vi "SetCurrentLimit.vi"(8 "error in (no error)":errorcluster, 9 "Current":dbl, 10 "Preset":enum16{"0", "1", "2", "3", ""}(ring), 11 "VISA resource name":refnum<visa-resource-name>) -> (0 "error out":errorcluster, 3 "VISA resource name out":refnum<visa-resource-name>)   [LabVIEW 2019, in "9103Series.lvlib"]
doc: "Set the output current limit of the power supply.\n\nPreset: Defines which preset memory to set.\nPreset Values: 3 - Default, 0 - A, 1 - B, 2 - C"
uses:
  <instrlib>/9103Series/9103Series.lvlib
panel:
  out "ok?":string
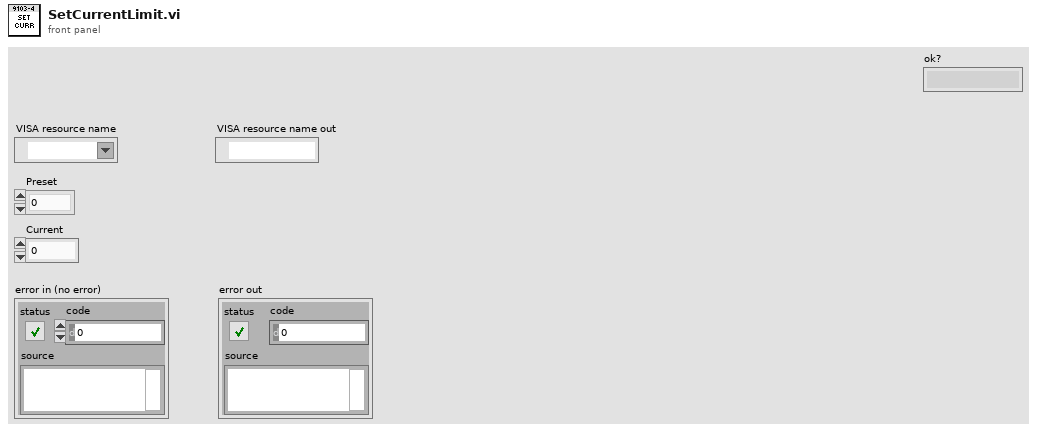
[diagram p1: front panel]
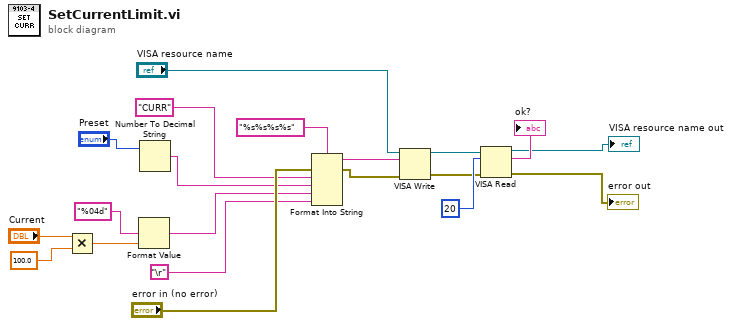
[diagram p0: block diagram]
diagram:
  n1 = Multiply(x="Current", y=100.0) -> (x*y=w17:dbl)
  n2 = Format Value(format string="%04d", value (0)=w17) -> (output string=w2:string)  [unwired: 1 in]
  n3 = Number To Decimal String(number="Preset") -> (decimal integer string=w3:string)  [unwired: 1 in]
  n4 = Format Into String(format string="%s%s%s%s", error in="error in (no error)", "CURR" ("string"), w3, w2, "\r") -> (resulting string=w8:string, error out=w7:errorcluster)  [unwired: 1 in]
  n5 = VISA Write(VISA resource name="VISA resource name", write buffer=w8, error in (no error)=w7) -> (VISA resource name out=w10:refnum<visa-resource-name>, error out=w9:errorcluster)  [unwired: 1 out]
  n6 = VISA Read(VISA resource name=w10, byte count=u32 20, error in (no error)=w9) -> (VISA resource name out=→"VISA resource name out":refnum<visa-resource-name>, read buffer=→"ok?":string, error out=→"error out":errorcluster)  [unwired: 1 out]
